vi "Set_Amplitude.vi"(7 "Menu Ring 2":u16(ring) items=["Channel 1", "Channel 2"], 9 "Amplitude":dbl=1.0, 11 "VISA resource name":refnum<visa-resource-name>="USB0::0x0699::0x0347::C036837::INSTR") -> (3 "VISA resource name out":refnum<visa-resource-name>)   [LabVIEW 2011]
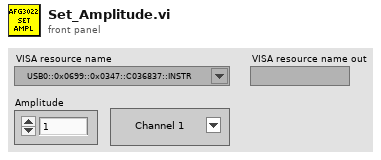
[diagram p1: front panel]
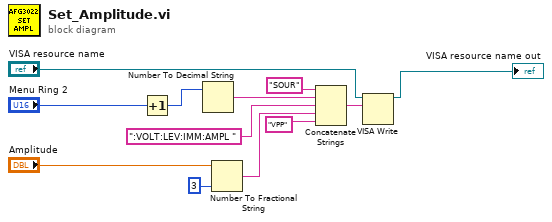
[diagram p0: block diagram]
diagram:
  n1 = Increment(x="Menu Ring 2") -> (x+1=w3:u16)
  n2 = Number To Decimal String(number=w3) -> (decimal integer string=w4:string)  [unwired: 1 in]
  n3 = Number To Fractional String(number="Amplitude", precision (6)=i16 3) -> (F-format string=w8:string)  [unwired: 2 in]
  n4 = Concatenate Strings("SOUR" ("string"), w4, ":VOLT:LEV:IMM:AMPL " ("string"), w8, "VPP" ("string")) -> (w9:string)
  n5 = VISA Write(VISA resource name="VISA resource name", write buffer=w9) -> (VISA resource name out=→"VISA resource name out":refnum<visa-resource-name>)  [unwired: 1 in, 2 out]
